vi "Get Joystick Values.vi"(8 "error in (no error)":errorcluster, 11 "Joysticks in":refnum<class "Joysticks.lvclass">) -> (0 "error out":errorcluster, 2 "Joystick Data":T1, 3 "Joysticks out":refnum<class "Joysticks.lvclass">)   [LabVIEW 2018, in "Joysticks.lvlib" / "Joysticks.lvclass"]
doc: "Use this method to get the joystick values in a cluster you can use for your application.\n\nModify the Type Def that this VI resturns to fit the controls needed for the robot."
uses:
  Joysticks.lvclass
  Controls/JoystickData.ctl
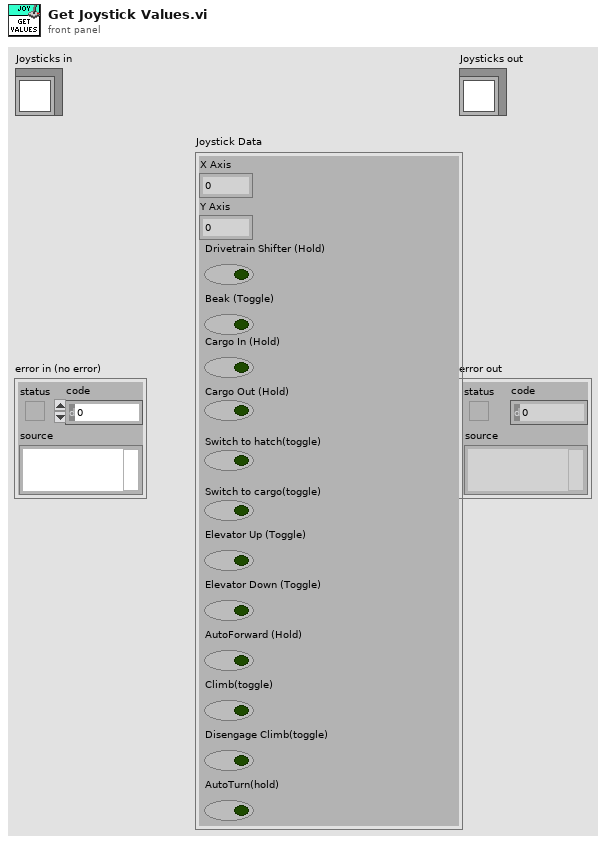
[diagram p1: front panel]
types:
  T1 = typedef "Joysticks.lvlib/Joysticks.lvclass/JoystickData.ctl" = cluster{"X Axis":dbl, "Y Axis":dbl, "Drivetrain Shifter (Hold)":bool, "Beak (Toggle)":bool, "Cargo In (Hold)":bool, "Cargo Out (Hold)":bool, "Switch to hatch(toggle)":bool, "Switch to cargo(toggle)":bool, "Elevator Up (Toggle)":bool, "Elevator Down (Toggle)":bool, "AutoForward (Hold)":bool, "Climb(toggle)":bool, "Disengage Climb(toggle)":bool, "AutoTurn(hold)":bool}
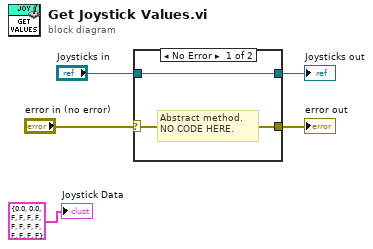
[diagram p0: block diagram]
diagram:
  n1 = case shown="No Error" "error in (no error)" {
    selector: "error in (no error)" -> [w6 w9]
    tunnel: [w6 w9] -> w4
    tunnel: [w7 w8] -> w2
    tunnel: "Joysticks in" -> [w7 w8]
    frame No Error {
      # "Abstract method.\nNO CODE HERE."
    }
    frame Error {
    }
  }
  "error out" <- w4
  "Joysticks out" <- w2
  "Joystick Data" <- T1 {"X Axis"=0.0, "Y Axis"=0.0, "Drivetrain Shifter (Hold)"=FALSE, "Beak (Toggle)"=FALSE, "Cargo In (Hold)"=FALSE, "Cargo Out (Hold)"=FALSE, "Switch to hatch(toggle)"=FALSE, "Switch to cargo(toggle)"=FALSE, "Elevator Up (Toggle)"=FALSE, "Elevator Down (Toggle)"=FALSE, "AutoForward (Hold)"=FALSE, "Climb(toggle)"=FALSE, "Disengage Climb(toggle)"=FALSE, "AutoTurn(hold)"=FALSE} ("Joystick Data")
